vi "NI9263_driver_RampWave.vi"(5 "Number of Samples":i32=1000, 6 "METHOD":T1, 7 "Sample Rate":dbl=1000.0, 8 "error in (no error)":errorcluster, 9 "End":dbl=1.0 format="%0.2p", 10 "Start":dbl format="%0.2p", 11 "Channels NI9263":tag="Dev1/ao0") -> (0 "error out":errorcluster, 3 "Waveform Graph":waveform(dbl)(graph))   [LabVIEW 2020]
uses:
  TYPEDEF/NI9263_TD_Method.ctl
  TYPEDEF/NI9263_TD_SetWave.ctl
  <vilib>/DAQmx/write.llb/DAQmx Write (Analog 1D Wfm NChan NSamp).vi
  <vilib>/DAQmx/create/channels.llb/DAQmx Create Channel (AO-Voltage-Basic).vi
  <vilib>/DAQmx/configure/timing.llb/DAQmx Timing (Sample Clock).vi
  <vilib>/DAQmx/miscellaneous.llb/DAQmx Fill In Error Info.vi
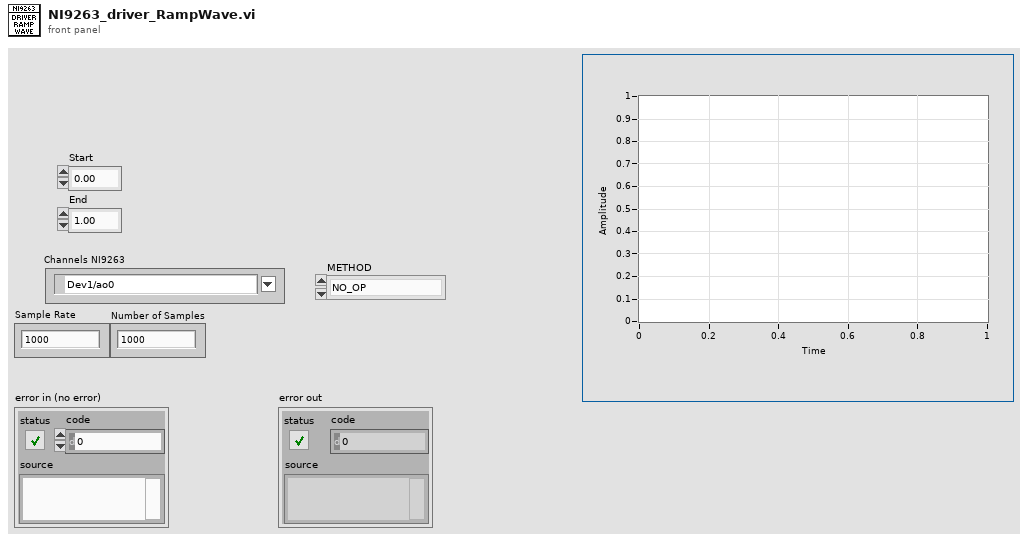
[diagram p1: front panel]
types:
  T1 = typedef "NI9263_TD_Method.ctl" = enum16{"NO_OP", "INIT", "SET", "GET", "CLOSE"}
  T2 = typedef "NI9263_TD_SetWave.ctl" = enum16{"RAMP"}
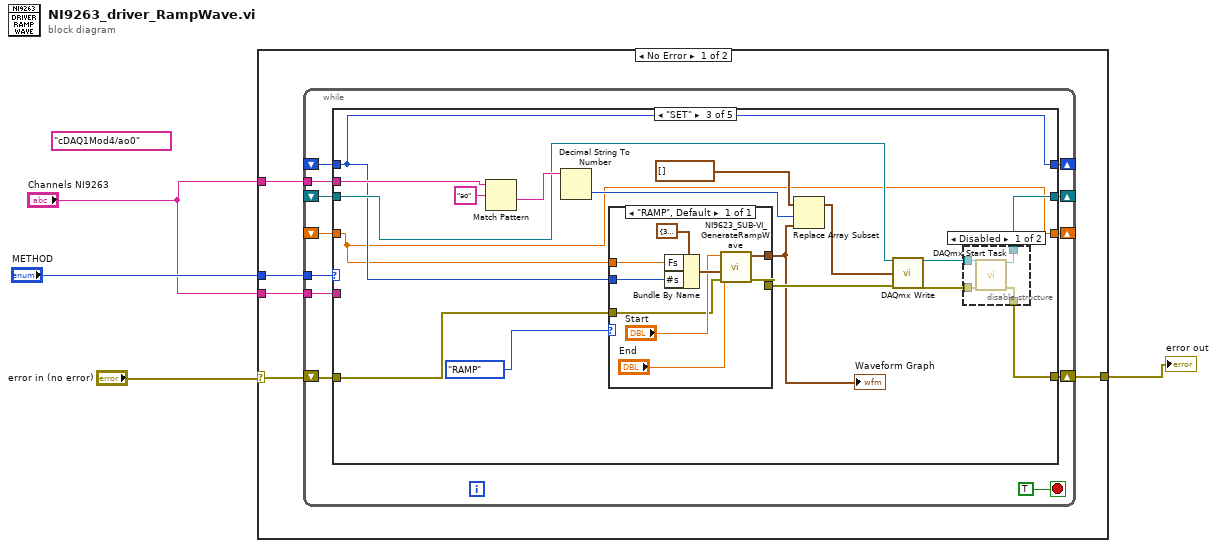
[diagram p0: block diagram]
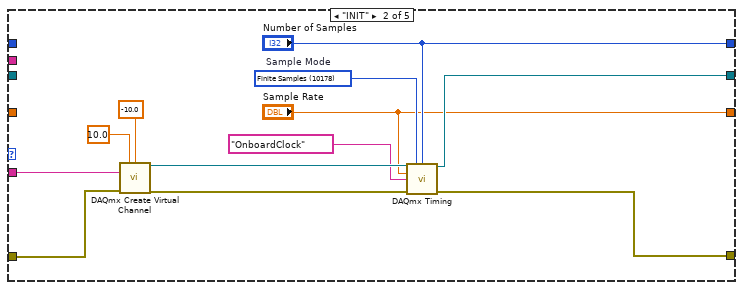
[diagram p3: hidden frame]
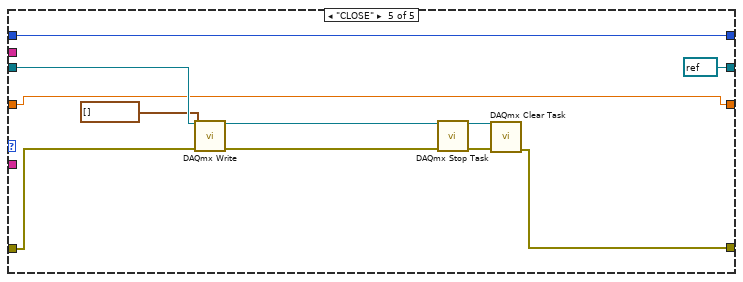
[diagram p6: hidden frame]
diagram:
  (unwired) tag "cDAQ1Mod4/ao0" ("physical channels")
  n1 = case shown="No Error" "error in (no error)" {
    selector: "error in (no error)" -> [w9 w85]
    tunnel: "METHOD" -> [w8 _]
    tunnel: "Channels NI9263" -> [w7 _]
    tunnel: [w6 w85] -> w2
    tunnel: "Channels NI9263" -> [w5 _]
    frame No Error {
      n2 = while {
        tunnel: w8 -> [w20]
        tunnel: w7 -> [w18]
        shift-right: [w17] -> _
        shift-left: _ -> [w16]
        shift-right: [w15] -> w6
        shift-left: w9 -> [w19]
        tunnel: w5 -> [w14]
        shift-right: [w13] -> _
        shift-left: _ -> [w12]
        shift-right: [w11] -> _
        shift-left: _ -> [w10]
        stop <- TRUE stop-if-true
        n3 = case shown="\"SET\"" w20 {
          tunnel: w19 -> [w24 w30 w40 w72 w76]
          tunnel: w18 -> [_ w29 _ _ _]
          tunnel: [w25 w37 w50 w73 refnum<k21> refnum ("task out")] -> w17
          tunnel: w16 -> [w25 _ w41 w73 w82]
          tunnel: [w24 w28 w49 w72 w79] -> w15
          tunnel: w14 -> [_ _ w45 _ _]
          tunnel: [w23 "Number of Samples" w39 w71 w75] -> w13
          tunnel: w12 -> [w23 _ w39 w71 w75]
          tunnel: [w22 "Sample Rate" w38 w70 w74] -> w11
          tunnel: w10 -> [w22 _ w38 w70 w74]
          frame "NO_OP", Default {
          }
          frame "INIT" {
            w36 = 10178 items=["Finite Samples"=10178, "Continuous Samples"=10123, "Hardware Timed Single Point"=12522]  # Sample Mode
            n4 = call-poly <vilib>:"DAQmx Create Virtual Channel.vi"("maximum value"=10.0 ("Max Voltage"), "minimum value"=-10.0 ("Min Voltage"), "physical channels"=w29, "error in"=w30) -> ("task out"=w34:refnum<k21>, "error out"=w35:errorcluster)  [unwired: 10 in]
            n5 = call-poly <vilib>:"DAQmx Timing.vi"("task/channels in"=w34, "sample mode"=w36, "samples per channel"="Number of Samples", "rate"="Sample Rate", "source"=tag "OnboardClock" ("Sample Clock Source"), "error in"=w35) -> ("task out"=w37:refnum<k21>, "error out"=w28:errorcluster)  [unwired: 8 in]
          }
          frame "SET" {
            n6 = Match Pattern(string=w45, regular expression="ao") -> (after substring=w44:string)  [unwired: 1 in, 3 out]
            n7 = Decimal String To Number(string=w44) -> (number=w43:i32)  [unwired: 2 in, 1 out]
            n8 = case shown="\"RAMP\", Default" NI9263_TD_SetWave."RAMP" ("SET_WAVE") {
              tunnel: [w67] -> w42
              tunnel: [w66] -> w53
              tunnel: w40 -> [w63]
              tunnel: w39 -> [w62]
              tunnel: w38 -> [w61]
              frame "RAMP", Default {
                n9 = Bundle By Name(cluster=cluster{"Fs":dbl, "#s":dbl} {"Fs"=300.0, "#s"=2000.0} ("sampling info"), "Fs"=w61, "#s"=w62) -> (w68:cluster{"Fs":dbl, "#s":dbl})
                n10 = call "NI9623_SUB-VI_GenerateRampWave.vi"("error in (no error)"=w63, "sampling info"=w68, "End"="End", "Start"="Start") -> ("error out"=w66:errorcluster, "signal out"=w67:waveform(dbl))  [unwired: 6 in]
              }
            }
            "Waveform Graph" <- w42
            n11 = Replace Array Subset(array=waveform(dbl)[] [] ("data"), new element=w42, index=w43) -> (w47:waveform(dbl)[])
            n12 = call-poly <vilib>:"DAQmx Write.vi"("task/channels in"=w41, "data"=w47, "error in"=w53) -> ("task out"=w51:refnum<k21>, "error out"=w52:errorcluster)  [unwired: 10 in, 1 out]
            n13 = disable-structure shown="Disabled" {
              disable-tunnel: w52 -> [w58 w59]
              disable-tunnel: w51 -> [w57 w60]
              disable-tunnel: [w56 w60] -> w50
              disable-tunnel: [w55 w59] -> w49
              frame Disabled {
                n14 = call <vilib>:"DAQmx Start Task.vi"("task/channels in"=w57, "error in"=w58) -> ("task out"=w56:refnum<k21>, "error out"=w55:errorcluster)  [unwired: 12 in]
              }
              frame Enabled {
              }
            }
          }
          frame "GET" {
          }
          frame "CLOSE" {
            n15 = call-poly <vilib>:"DAQmx Write.vi"("task/channels in"=w82, "data"=waveform(dbl)[] [], "error in"=w76) -> ("task out"=w81:refnum<k21>, "error out"=w80:errorcluster)  [unwired: 10 in, 1 out]
            n16 = call <vilib>:"DAQmx Stop Task.vi"("task/channels in"=w81, "error in"=w80) -> ("task out"=w83:refnum<k21>, "error out"=w84:errorcluster)  [unwired: 12 in]
            n17 = call <vilib>:"DAQmx Clear Task.vi"("task in"=w83, "error in"=w84) -> ("error out"=w79:errorcluster)  [unwired: 13 in]
          }
        }
      }
    }
    frame Error {
    }
  }
  "error out" <- w2
